vi "Find_float.vi"() -> ()   [LabVIEW 2018]
panel:
  out "*(type *) &x 4":dbl
  out "*(type *) &x 3":dbl
  out "*(type *) &x 2":dbl
  out "*(type *) &x":dbl
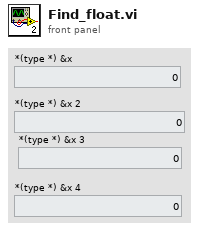
[diagram p1: front panel]
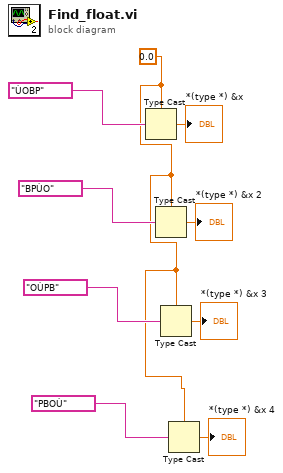
[diagram p0: block diagram]
diagram:
  w1 = sgl 0.0
  n1 = Type Cast(type=w1, x="ÙOBP") -> (*(type *) &x=→"*(type *) &x":sgl)
  n2 = Type Cast(type=w1, x="BPÙO") -> (*(type *) &x=→"*(type *) &x 2":sgl)
  n3 = Type Cast(type=w1, x="OÙPB") -> (*(type *) &x=→"*(type *) &x 3":sgl)
  n4 = Type Cast(type=w1, x="PBOÙ") -> (*(type *) &x=→"*(type *) &x 4":sgl)
